vi "温湿度参数配置.vi"() -> ()   [LabVIEW 2016, in "环境动力监测库.lvlib"]
panel:
  in  "高温告警启用":bool caption="高温告警"
  in  "湿度下限告警点":dbl
  in  "湿度上限告警点":dbl
  in  "室温下限告警点":dbl
  in  "室温上限告警点":dbl
  in  "模拟量配置":bool
  # "温湿度参数配置"
  # "℃"
  # "℃"
  # "%"
  # "%"
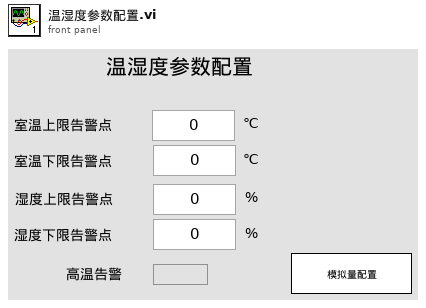
[diagram p1: front panel]
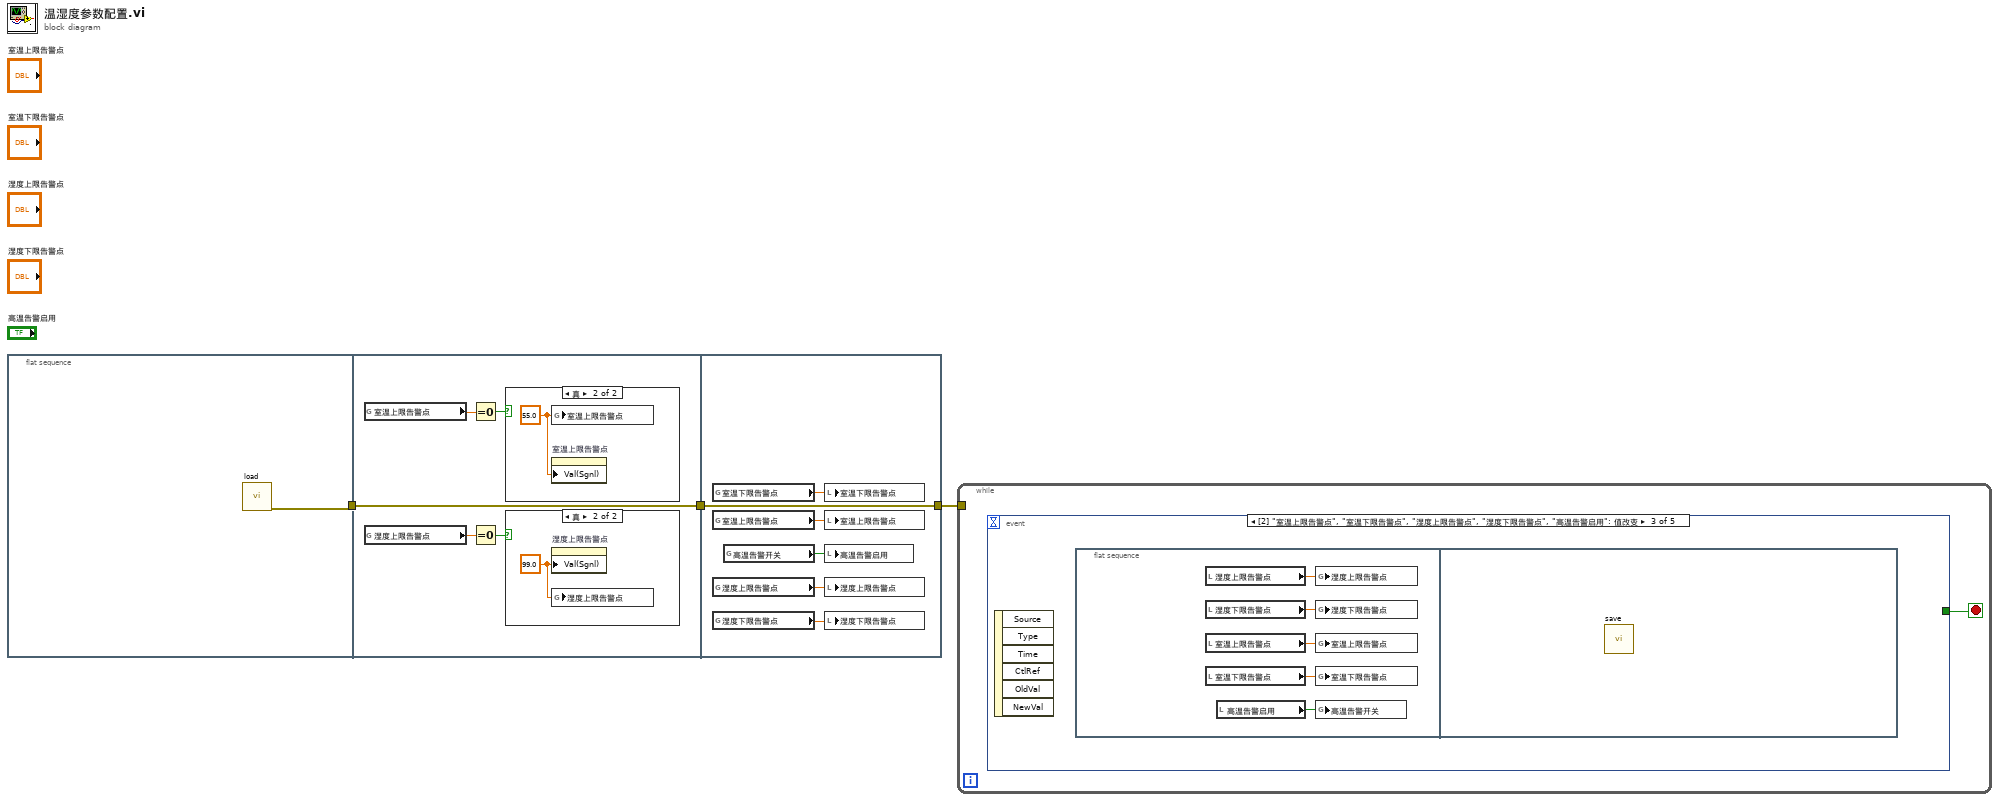
[diagram p0: block diagram]
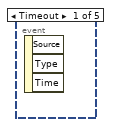
[diagram p4: hidden frame]
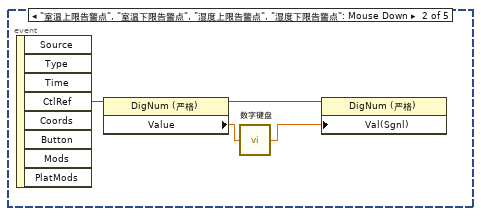
[diagram p5: hidden frame]
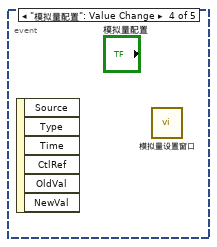
[diagram p6: hidden frame]
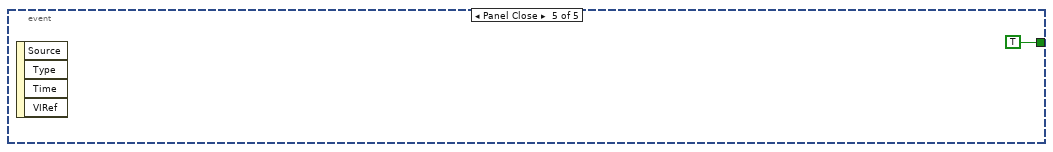
[diagram p7: hidden frame]
diagram:
  n1 = flat-sequence {
    tunnel: [w4] -> w2
    tunnel: w2 -> [w9]
    tunnel: [w9] -> w1
    tunnel: [w17] -> w3
    tunnel: w1 -> [w17]
    frame #0 {
      n2 = call "load.vi"() -> ("error out"=w4:errorcluster)  [unwired: 11 in]
    }
    frame #1 {
      n3 = global read "断电保存全局变量.vi" "室温上限告警点"() -> (w8:dbl)
      n4 = global read "断电保存全局变量.vi" "湿度上限告警点"() -> (w6:dbl)
      n5 = Equal To 0?(x=w8) -> (x = 0?=w7:bool)
      n6 = Equal To 0?(x=w6) -> (x = 0?=w5:bool)
      n7 = case shown="真" w7 {
        frame False {
        }
        frame True {
          w11 = 55.0 ("室温上限告警点")
          n8 = global write "断电保存全局变量.vi" "室温上限告警点"(w11) -> ()
          n9 = property on="室温上限告警点" class="DigNum (严格)"("Val(Sgnl)"=w11) -> ()  [unwired: 2 in, 2 out]
        }
      }
      n10 = case shown="真" w5 {
        frame False {
        }
        frame True {
          w10 = 99.0 ("室温上限告警点")
          n11 = property on="湿度上限告警点" class="DigNum (严格)"("Val(Sgnl)"=w10) -> ()  [unwired: 2 in, 2 out]
          n12 = global write "断电保存全局变量.vi" "湿度上限告警点"(w10) -> ()
        }
      }
    }
    frame #2 {
      n13 = global read "断电保存全局变量.vi" "室温下限告警点"() -> (w16:dbl)
      n14 = global read "断电保存全局变量.vi" "室温上限告警点"() -> (w15:dbl)
      n15 = global read "断电保存全局变量.vi" "湿度上限告警点"() -> (w13:dbl)
      n16 = global read "断电保存全局变量.vi" "湿度下限告警点"() -> (w14:dbl)
      n17 = global read "断电保存全局变量.vi" "高温告警开关"() -> (w12:bool)
      n18 = local write "室温下限告警点"(w16) -> ()
      n19 = local write "室温上限告警点"(w15) -> ()
      n20 = local write "高温告警启用"(w12) -> ()
      n21 = local write "湿度上限告警点"(w13) -> ()
      n22 = local write "湿度下限告警点"(w14) -> ()
    }
  }
  n23 = while {
    tunnel: w3 -> [_]
    stop <- w18 stop-if-true
    n24 = event shown="[2] \"室温上限告警点\", \"室温下限告警点\", \"湿度上限告警点\", \"湿度下限告警点\", \"高温告警启用\": 值改变" {
      selector: _ -> [_ _ _ _ _]
      dyn-events: _ -> [_ _ _ _ _]
      timeout: _ -> [_ _ _ _ _]
      tunnel: [_ _ _ _ TRUE] -> w18
      event Timeout {
        n25 = event-data() -> ()  [unwired: 1 in, 3 out]
      }
      event "室温上限告警点", "室温下限告警点", "湿度上限告警点", "湿度下限告警点": Mouse Down {
        n26 = event-data() -> ("CtlRef"=w19:refnum<vi>)  [unwired: 1 in, 7 out]
        n27 = property class="DigNum (严格)"(reference=w19) -> (reference out=w21:refnum<vi>, "Value"=w22:dbl)  [unwired: 1 in, 1 out]
        n28 = call "数字键盘.vi"("OldNumber"=w22) -> ("NewNumber"=w20:sgl)
        n29 = property class="DigNum (严格)"(reference=w21, "Val(Sgnl)"=w20) -> ()  [unwired: 1 in, 2 out]
      }
      event "室温上限告警点", "室温下限告警点", "湿度上限告警点", "湿度下限告警点", "高温告警启用": Value Change {
        n30 = event-data() -> ()  [unwired: 1 in, 6 out]
        n31 = flat-sequence {
          frame #0 {
            n32 = local read "湿度上限告警点"() -> (w27:dbl)
            n33 = local read "湿度下限告警点"() -> (w26:dbl)
            n34 = local read "室温上限告警点"() -> (w25:dbl)
            n35 = local read "室温下限告警点"() -> (w24:dbl)
            n36 = local read "高温告警启用"() -> (w23:bool)
            n37 = global write "断电保存全局变量.vi" "湿度上限告警点"(w27) -> ()
            n38 = global write "断电保存全局变量.vi" "湿度下限告警点"(w26) -> ()
            n39 = global write "断电保存全局变量.vi" "室温上限告警点"(w25) -> ()
            n40 = global write "断电保存全局变量.vi" "室温下限告警点"(w24) -> ()
            n41 = global write "断电保存全局变量.vi" "高温告警开关"(w23) -> ()
          }
          frame #1 {
            n42 = call "save.vi"() -> ()  [unwired: 11 in, 1 out]
          }
        }
      }
      event "模拟量配置": Value Change {
        n43 = event-data() -> ()  [unwired: 1 in, 6 out]
        n44 = call "模拟量设置窗口.vi"() -> ()  [unwired: 12 in]
      }
      event Panel Close {
        n45 = event-data() -> ()  [unwired: 1 in, 4 out]
      }
    }
  }
